vi "Initialize.vi"(11 "Graph in":refnum<class "Graph.lvclass">) -> (3 "Graph out":refnum<class "Graph.lvclass">)   [LabVIEW 2024, in "Graph.lvclass"]
uses:
  Graph.lvclass
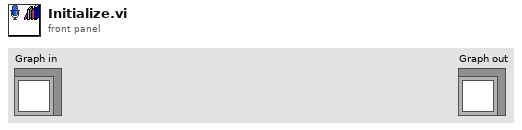
[diagram p1: front panel]
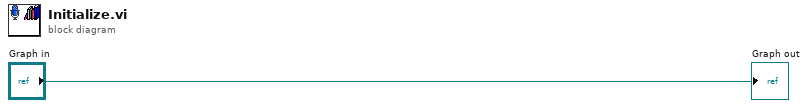
[diagram p0: block diagram]
diagram:
  "Graph out" <- "Graph in"
